vi "CVT Bool IndexRead.vi"(3 "error in (no error)":errorcluster, 5 "Tag Index":i32) -> (0 "error out":errorcluster, 1 "Value":bool)   [LabVIEW 2014, in "QwaveSys Raspberry Pi Library.lvlib"]
uses:
  _SubVIs/TypeDefs/cvt_MemBlock Methods.ctl
  QwaveSys Raspberry Pi Library.lvlib
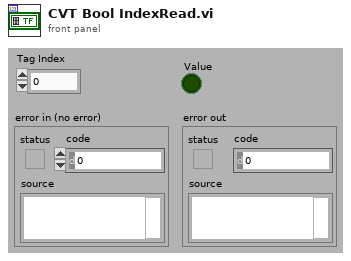
[diagram p1: front panel]
types:
  T1 = typedef "QwaveSys Raspberry Pi Library.lvlib/cvt_MemBlock Methods.ctl" = enum16{"init", "read", "readall", "write"}
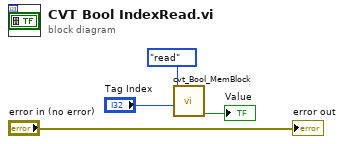
[diagram p0: block diagram]
diagram:
  n1 = call "cvt_Bool_MemBlock.vi"("Index"="Tag Index", "Method"=cvt_MemBlock_Methods."read") -> ("Value"=→"Value":bool)  [unwired: 2 in, 7 out]
  "error out" <- "error in (no error)"
